vi "2100_Average HV meas under Load.vi"(7 "Num_Iterations_Per_Load_Step":i32=20, 8 "Error In":errorcluster, 10 "voltage measurements":dbl[](array[numeric])=[41.400019787154584, 41.491719884993515, 41.449526588441856, 41.407333291890204, 41.36626514991326, 41.397206900717805, 41.46246586605103, 41.421960301361445, 41.38032958209715, 41.350512985867304, 41.48159349382112, 41.4377124654074, 41.39383143699368, 41.35220071772937, 41.448401433867154, 41.45065174301657, 41.40902102375227, 41.365702572625906, 41.349387831292596, 41.47034194807401, 41.42814865152235, 41.384267623108634, 41.34151174926962, 41.47259225722343, 41.44052535184417, 41.39889463257987, 41.35276329501673, 41.397206900717805, 41.458527825039546, 41.417459683062596, 41.37189092278681, 41.33082278080987, 41.47990576195905, 41.43714988812004, 41.394394014281026, 41.35220071772937, 41.391581127844255, 41.45627751589013, 41.41127133290169, 41.369640613637394, 41.33194793538458, 41.47202967993607, 41.429273806097065, 41.38764308683277, 41.34657494485582, 41.47371741179815, 41.44727627929244, 41.40508298274078, 41.36457741805119, 41.350512985867304, 41.350512985867304, 41.17555144949977, 41.243060723982424, 41.27569020664904, 41.266126392763994, 41.25993804260308, 41.29931845271796, 41.317320925913336, 41.247561342281266, 41.273439897499614, 41.29650556628119, 41.30494422559152, 41.243060723982424, 41.27569020664904, 41.297068143568545, 41.31338288490185, 41.27906567037317, 41.238560105683575, 41.27456505207432, 41.29313010255706, 41.30944484389036, 41.25825031074102, 41.26556381547664, 41.29031721612028, 41.27794051579846, 41.243060723982424, 41.27625278393639, 41.29481783441912, 41.310007421177716, 41.289754638832925, 41.23124660094796, 41.26893927920077, 41.29144237069499, 41.30156876186739, 41.24249814669507, 41.257687733453665, 41.28412886595937, 41.298193298143254, 41.31338288490185, 41.26556381547664, 41.231809178235316, 41.26837670191342, 41.286941752396146, 41.30156876186739, 41.307194534740944, 41.24474845584449, 41.273439897499614, 41.297068143568545, 41.31113257575243, 41.28581659782144, 41.23912268297094, 41.27794051579846, 41.29594298899383, 41.30944484389036, 41.32069638963747, 41.25374969244218, 41.2610631971778, 41.288629484258216, 41.30494422559152, 41.31113257575243, 41.238560105683575, 41.26162577446515, 41.2875043296835, 41.3077571120283, 41.31450803947656, 41.24924907414333, 41.262188351752506, 41.289754638832925, 41.30606938016623, 41.310007421177716, 41.227308559936475, 41.25825031074102, 41.28581659782144, 41.29875587543061, 41.31394546218921, 41.27456505207432, 41.24362330126978, 41.27681536122375, 41.298193298143254, 41.311695153039786, 41.27850309308581, 41.257687733453665, 41.2875043296835, 41.305506802878874, 41.27794051579846, 41.25712515616631, 41.28581659782144, 41.304381648304165, 41.30888226660301, 41.24418587855713, 41.274002474786975, 41.298193298143254, 41.31394546218921, 41.310007421177716, 41.238560105683575, 41.26950185648813, 41.29144237069499, 41.30831968931565, 41.285254020534076], 11 "HV_Load_Steps_uA":dbl[](array[numeric])=[0.0, 2.0, 0.0, 4.0, 0.0, 6.0, 0.0, 8.0, 0.0, 10.0, 0.0, 12.0, 0.0, 14.0, 0.0, 16.0, 0.0, 20.0, 0.0] format="%#_6p") -> (0 "Error Out":errorcluster, 3 "Avg_Meas_HV":dbl[](array[numeric]))   [LabVIEW 2013]
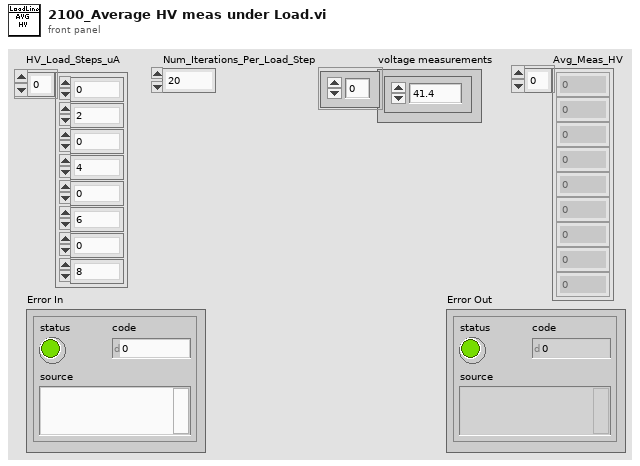
[diagram p1: front panel]
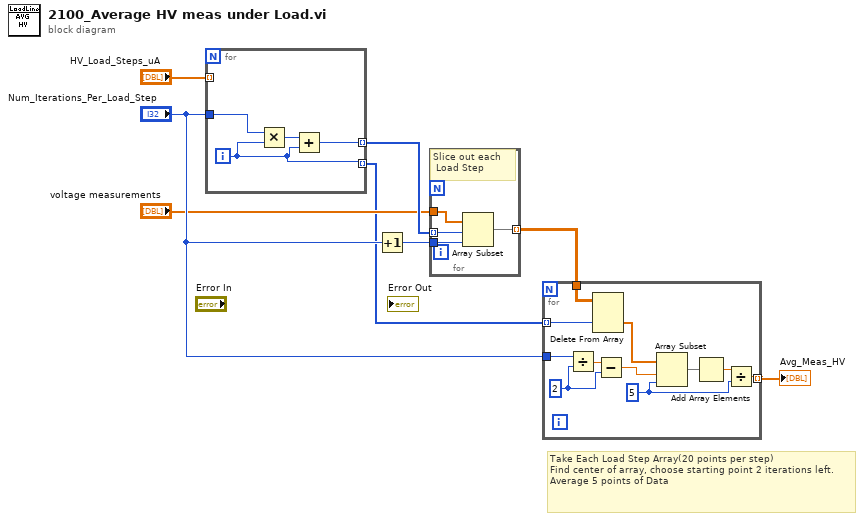
[diagram p0: block diagram]
diagram:
  # "Take Each Load Step Array(20 points per step)\nFind center of array, choose starting point 2 iterations left.\nAverage 5 points of Data"
  n1 = for {
    tunnel: "HV_Load_Steps_uA" -> [_] mode=indexing
    tunnel: "Num_Iterations_Per_Load_Step" -> [w12]
    tunnel: [w10] -> w8 mode=indexing
    tunnel: [w9] -> w1 mode=indexing
    i -> [w9]
    n2 = Multiply(x=w12, y=w9) -> (x*y=w11:i32)
    n3 = Add(x=w11, y=w9) -> (x+y=w10:i32)
  }
  n4 = Increment(x="Num_Iterations_Per_Load_Step") -> (x+1=w7:i32)
  n5 = for {
    tunnel: w8 -> [w15] mode=indexing
    tunnel: "voltage measurements" -> [w16]
    tunnel: w7 -> [w14]
    tunnel: [w13] -> w6 mode=indexing
    # "Slice out each\n Load Step"
    n6 = Array Subset(array=w16, index=w15, length=w14) -> (w13:dbl[])
  }
  n7 = for {
    tunnel: w6 -> [w27]
    tunnel: "Num_Iterations_Per_Load_Step" -> [w26]
    tunnel: [w18] -> w2 mode=indexing
    tunnel: w1 -> [w17] mode=indexing
    w19 = 5 ("length")
    w24 = 2 ("y")
    n8 = Divide(x=w26, y=w24) -> (x/y=w25:dbl)
    n9 = Delete From Array(array=w27, index (row)=w17) -> (deleted portion=w22:dbl[])  [unwired: 2 in, 1 out]
    n10 = Subtract(x=w25, y=w24) -> (x-y=w23:dbl)
    n11 = Array Subset(array=w22, index=w23, length=w19) -> (w21:dbl[])
    n12 = Add Array Elements(numeric array=w21) -> (sum=w20:dbl)
    n13 = Divide(x=w20, y=w19) -> (x/y=w18:dbl)
  }
  "Avg_Meas_HV" <- w2
